vi "Create All Message Queues.vi"(8 "error in (no error)":errorcluster, 11 "initialization messages":string[](array[string])) -> (0 "error out":errorcluster, 3 "Message Queues out":T1)   [LabVIEW 2019, in "HLA Custom Device Engine.lvlib" / "Message Queue.lvlib"]
doc: "This VI creates and initializes all the message queues for your application. If your application requires more than one message queue, right-click the \"Message Queues\" constant above and select Open Type Def. Add the new Message Queue(s) to the type definition, then initialize them in this VI."
uses:
  Message Queue.lvlib
  All Message Queues.ctl
  Message Cluster.ctl
  Enqueue Message (Single).vi
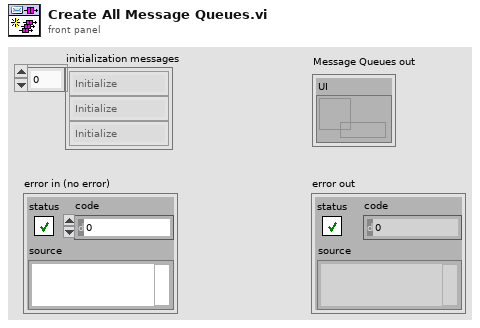
[diagram p1: front panel]
types:
  T1 = typedef "HLA Custom Device Engine.lvlib/Message Queue.lvlib/All Message Queues.ctl" = cluster{"UI":refnum<queue>}
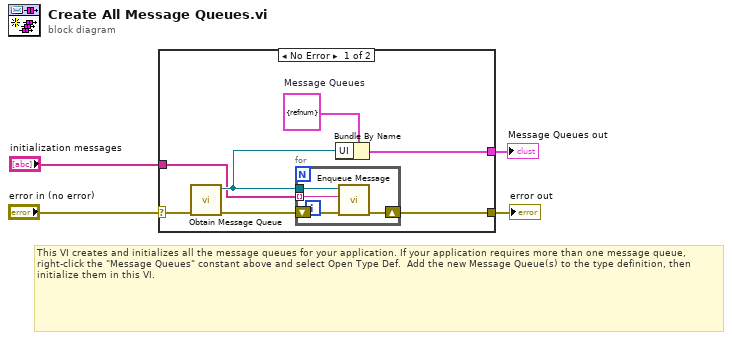
[diagram p0: block diagram]
diagram:
  # "This VI creates and initializes all the message queues for your application. If your application requires more than one message queue, right-click the \"Message Queues\" constant above and select Open Type Def.  Add the new Message Queue(s) to the type definition, then initialize them in this VI."
  n1 = case shown="No Error" "error in (no error)" {
    selector: "error in (no error)" -> [w8 w16]
    tunnel: [w11 w16] -> w4
    tunnel: [w9 _] -> w3
    tunnel: "initialization messages" -> [w5 _]
    frame No Error {
      w10 = T1 {"UI"=refnum}  # Message Queues
      n2 = call "Obtain Message Queue.vi"("error in (no error)"=w8) -> ("error out"=w7:errorcluster, "Message Queue"=w6:refnum<queue>)  [unwired: 9 in]
      n3 = for {
        tunnel: w6 -> [w13]
        tunnel: w5 -> [w12] mode=indexing
        shift-right: [w15] -> w11
        shift-left: w7 -> [w14]
        n4 = call-poly "Enqueue Message.vi"("error in (no error)"=w14, "Message"=w12, "Message Queue"=w13) -> ("error out"=w15:errorcluster)  [unwired: 7 in, 1 out]
      }
      n5 = Bundle By Name(cluster=w10, "UI"=w6) -> (w9:T1)
    }
    frame Error {
    }
  }
  "Message Queues out" <- w3
  "error out" <- w4
